vi "Project.SilentConnect.vi"(7 "Timeout (60000 ms)":u32=60000, 8 "Calibration File":path, 9 "Undeploy System Definition (F)":bool, 10 "System Definition File (.nivssdf)":path, 11 "Gateway IP Address (\"\": localhost)":string) -> (0 "error out":errorcluster)   [LabVIEW 2013, in "MiscHelperVIs.lvlib"]
uses:
  MiscHelperVIs.lvlib
  <vilib>/NI Veristand/Execution/Workspace/NI_VS Workspace ExecutionAPI.lvlib
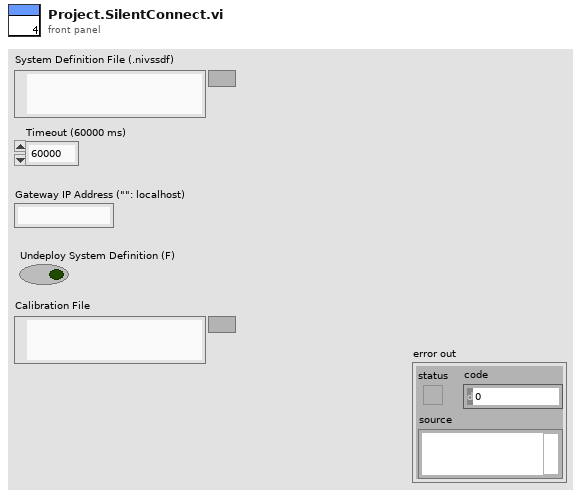
[diagram p1: front panel]
types:
  T1 = typedef "NI_VS Workspace ExecutionAPI.lvlib/WorkspaceAPI.ctl" = refnum<k24>
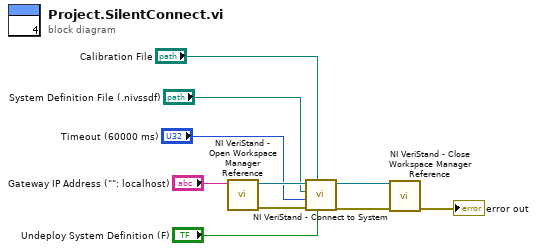
[diagram p0: block diagram]
diagram:
  n1 = call <vilib>:"NI VeriStand - Open Workspace Manager Reference.vi"("Gateway IP Address (\"\": localhost)"="Gateway IP Address (\"\": localhost)") -> ("error out"=w10:errorcluster, "WorkspaceManager"=w8:T1)  [unwired: 9 in]
  n2 = call <vilib>:"NI VeriStand - Connect to System.vi"("Deploy System Definition (T)"="Undeploy System Definition (F)", "Calibration File"="Calibration File", "error in (no error)"=w10, "Timeout (60000 ms)"="Timeout (60000 ms)", "System Definition File (.nivssdf)"="System Definition File (.nivssdf)", "WorkspaceManager in"=w8) -> ("error out"=w6:errorcluster, "WorkspaceManager out"=w5:T1)  [unwired: 4 in]
  n3 = call <vilib>:"NI VeriStand - Close Workspace Manager Reference.vi"("error in (no error)"=w6, "WorkspaceManager"=w5) -> ("error out"=→"error out":errorcluster)  [unwired: 9 in]
